vi "POST (Multipart).vi"(6 "timeout":i32=10000, 7 "output file":path, 8 "error in":errorcluster, 9 "Multipart Post data":T1[](array[typedef]), 10 "url":string, 11 "http-method in":refnum<class "basic-http-client.lvclass">) -> (0 "error out":errorcluster, 2 "response":refnum<class "response.lvclass">, 3 "http-method out":refnum<class "basic-http-client.lvclass">)   [LabVIEW 2020, in "http.lvlib" / "basic-http-client.lvclass"]
uses:
  basic-http-client.lvclass
  response/response.lvclass
  <vilib>/httpClient/MultipartData.ctl
  basic-http-client.lvclass/basic-http-client.ctl
  <vilib>/httpClient/LabVIEWHTTPClient.lvlib
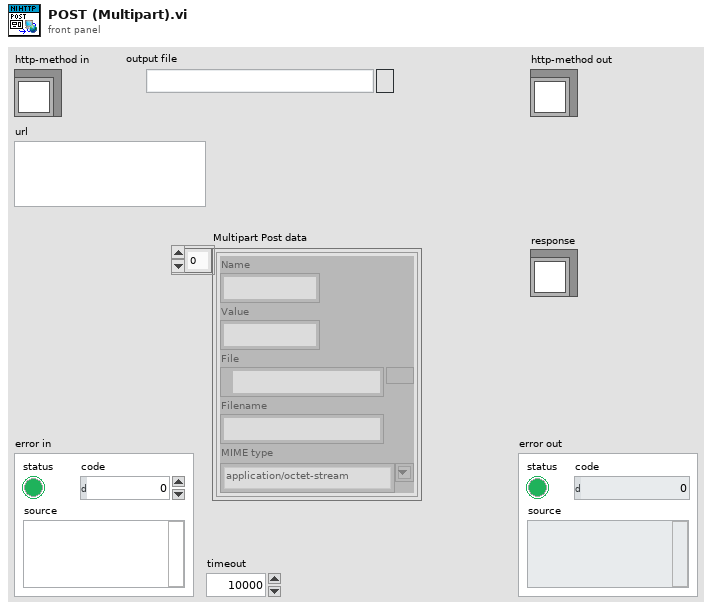
[diagram p1: front panel]
types:
  T1 = typedef "LabVIEWHTTPClient.lvlib/MultipartData.ctl" = cluster{"Name":string, "Value":string, "File":path, "Filename":string, "MIME type":string}
  T2 = typedef "LabVIEWHTTPClient.lvlib/ClientHandle.ctl" = refnum<k1>
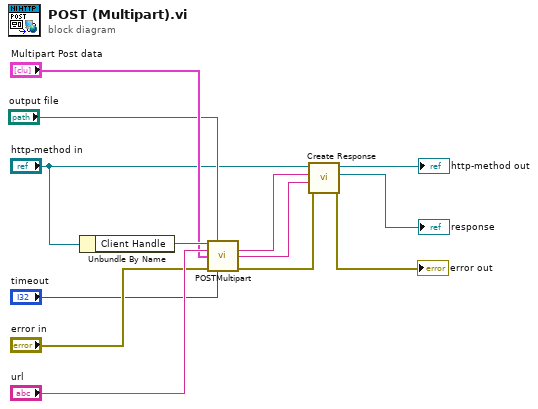
[diagram p0: block diagram]
diagram:
  n1 = Unbundle By Name("http-method in") -> ("Client Handle"=w13:T2)
  n2 = call <vilib>:"POSTMultipart.vi"("client handle"=w13, "output file"="output file", "url"="url", "data"="Multipart Post data", "error in (no error)"="error in", "timeout (10000)"="timeout") -> ("headers"=w5:string, "body"=w1:string, "error out"=w4:errorcluster)  [unwired: 6 in, 1 out]
  n3 = call-dynamic "Create Response.vi"("error in (no error)"=w4, "body"=w1, "headers"=w5, "http-client"="http-method in") -> ("error out"=→"error out":errorcluster, "response"=→"response":refnum<class "response.lvclass">, "http-client out"=→"http-method out":refnum<class "basic-http-client.lvclass">)  [unwired: 5 in]
